vi "DAQ2ANA Data Interface.vi"(8 "error in (no error)":errorcluster, 10 "DAQ2ANA":T1[](array[typedef]), 11 "Tree Ref":refnum<vi>) -> (0 "error out":errorcluster)   [LabVIEW 2016]
uses:
  Ctrls/PSVCH_All Channels.ctl
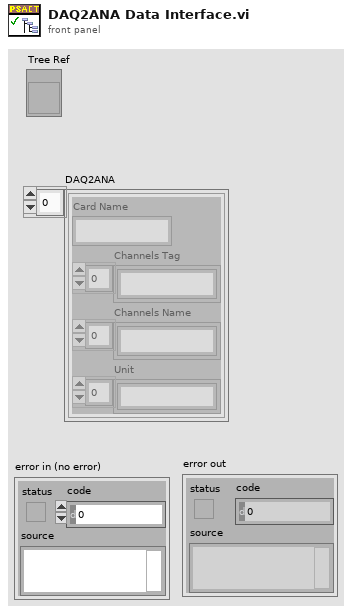
[diagram p1: front panel]
types:
  T1 = typedef "PSVCH_All Channels.ctl" = cluster{"Card Name":string, "Channels Tag":string[], "Channels Name":string[], "Unit":string[]}
  T2 = cluster{"Left Cell String":string, "Child Text":string[], "Child Tag":string, "Item Indent":i32, "Child Only?":bool, "Glyph Index":i32}
  T3 = cluster{"Left Cell String":string, "Child Text":string[], "Child Tag":string, "Item Indent":i32, "Child Only?":bool, "Glyph Index":i32}[]
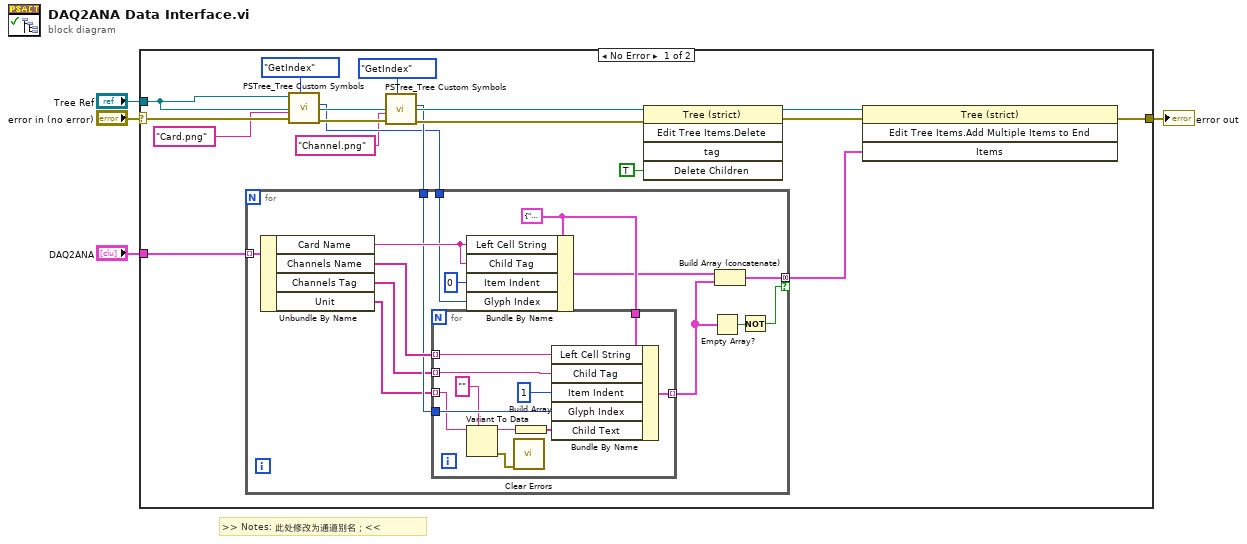
[diagram p0: block diagram]
diagram:
  # ">> Notes: 此处修改为通道别名；<<"
  n1 = case shown="No Error" "error in (no error)" {
    selector: "error in (no error)" -> [w15 w46]
    tunnel: "DAQ2ANA" -> [w17 _]
    tunnel: [w16 w46] -> w3
    tunnel: "Tree Ref" -> [w14 _]
    frame No Error {
      n2 = call "PSTree_Tree Custom Symbols.vi"("Operation"=enum16{"Register", "GetIndex"}."GetIndex", "error in (no error)"=w15, "PicName"="Card.png", "tree refnum"=w14) -> ("error out"=w10:errorcluster, "PicIndex"=w7:i32)  [unwired: 6 in]
      n3 = call "PSTree_Tree Custom Symbols.vi"("Operation"=enum16{"Register", "GetIndex"}."GetIndex", "error in (no error)"=w10, "PicName"="Channel.png") -> ("error out"=w9:errorcluster, "PicIndex"=w8:i32)  [unwired: 7 in]
      n4 = for {
        tunnel: w17 -> [w34] mode=indexing
        tunnel: w8 -> [w28]
        tunnel: w7 -> [w27]
        tunnel: [w24] -> w5 mode=concatenating if=w21
        w30 = T2 {"Left Cell String"="", "Child Text"=[], "Child Tag"="", "Item Indent"=0, "Child Only?"=FALSE, "Glyph Index"=0} ("Item")
        n5 = Unbundle By Name(w34) -> ("Card Name"=w33:string, "Channels Name"=w31:string[], "Channels Tag"=w26:string[], "Unit"=w25:string[])
        n6 = for {
          tunnel: w31 -> [w44] mode=indexing
          tunnel: w30 -> [w45]
          tunnel: [w42] -> w23 mode=indexing
          tunnel: w28 -> [w40]
          tunnel: w26 -> [w41] mode=indexing
          tunnel: w25 -> [w39] mode=indexing
          n7 = Variant To Data(type="", Variant=w39) -> (data=w37:string, error out=w35:errorcluster)  [unwired: 1 in]
          n8 = call <vilib>:"Clear Errors.vi"("error in (no error)"=w35) -> ()  [unwired: 5 in, 2 out]
          n9 = Build Array(w37) -> (w36:string[])
          n10 = Bundle By Name(cluster=w45, "Left Cell String"=w44, "Child Tag"=w41, "Item Indent"=1, "Glyph Index"=w40, "Child Text"=w36) -> (w42:T2)
        }
        n11 = Bundle By Name(cluster=w30, "Left Cell String"=w33, "Child Tag"=w33, "Item Indent"=0, "Glyph Index"=w27) -> (w29:T2)
        n12 = Empty Array?(array=w23) -> (empty?=w22:bool)
        n13 = Build Array (concatenate)(w29, w23) -> (w24:T3)
        n14 = Not(x=w22) -> (.not. x?=w21:bool)
      }
      n15 = invoke class="Tree (strict)" method="Edit Tree Items.Delete"(reference=w14, error in=w9, "Delete Children"=TRUE ("Delete Children?")) -> (reference out=w19:refnum<vi>, error out=w18:errorcluster)  [unwired: 2 in, 3 out]
      n16 = invoke class="Tree (strict)" method="Edit Tree Items.Add Multiple Items to End"(reference=w19, error in=w18, "Items"=w5) -> (error out=w16:errorcluster)  [unwired: 1 in, 3 out]
    }
    frame Error {
    }
  }
  "error out" <- w3
